vi "Disconnect.vi"(0 "reference in":refnum<class "Database_ODBC.lvclass">, 11 "error in (no error)":errorcluster) -> (4 "reference out":refnum<class "Database_ODBC.lvclass">, 15 "error out":errorcluster)   [LabVIEW 2019, in "Database_ODBC.lvclass"]
uses:
  Database_ODBC.lvclass
  Database_ODBC.lvclass/Database_ODBC.ctl
  <vilib>/addons/database/NI_Database_API.lvlib
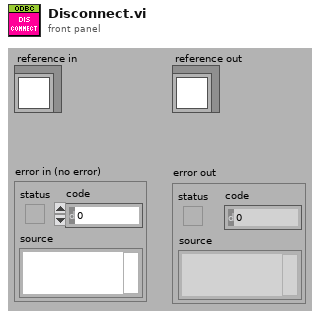
[diagram p1: front panel]
types:
  T1 = typedef "NI_Database_API.lvlib/Conn ObjectReference.ctl" = refnum<k1>
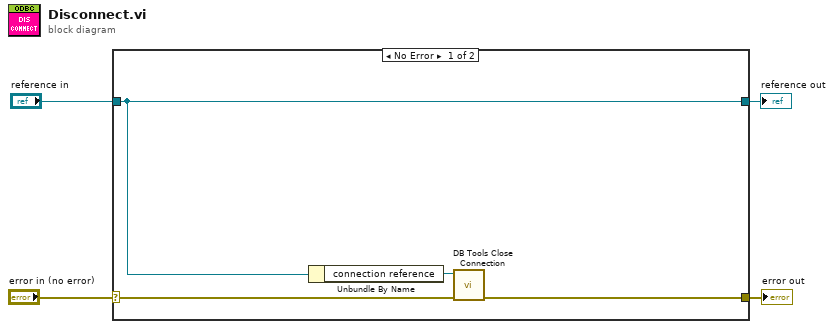
[diagram p0: block diagram]
diagram:
  n1 = case shown="No Error" "error in (no error)" {
    selector: "error in (no error)" -> [w8 w10]
    tunnel: [w5 w10] -> w3
    tunnel: [w7 w9] -> w1
    tunnel: "reference in" -> [w7 w9]
    frame No Error {
      n2 = Unbundle By Name(w7) -> ("connection reference"=w6:T1)
      n3 = call <vilib>:"DB Tools Close Connection.vi"("error in (no error)"=w8, "connection reference"=w6) -> ("error out"=w5:errorcluster)  [unwired: 5 in]
    }
    frame Error {
    }
  }
  "error out" <- w3
  "reference out" <- w1
